vi "write to descriptions.vi"(6 "comment":string, 7 "index":i32, 8 "error in":errorcluster, 9 "Y coords (in moter coordinate)":dbl, 10 "X coords (in moter coordinate)":dbl, 11 "Path of description file":path) -> (0 "error out":errorcluster, 3 "path out":path)   [LabVIEW 2017]
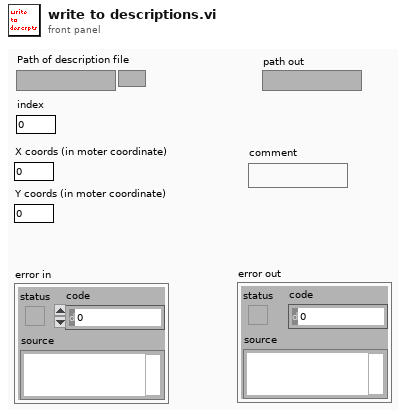
[diagram p1: front panel]
types:
  T1 = enum16{"open", "replace", "create", "open or create", "replace or create", "replace or create with confirmation"}
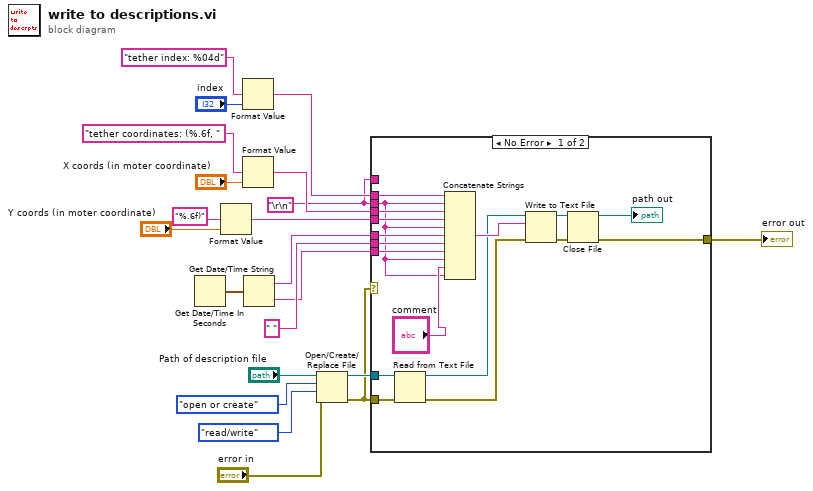
[diagram p0: block diagram]
diagram:
  w1 = "\r\n"
  n1 = Get Date/Time In Seconds() -> (seconds since 1Jan1904=w21:timestamp)
  n2 = Format Value(format string="%.6f)", value (0)="Y coords (in moter coordinate)") -> (output string=w12:string)  [unwired: 1 in]
  n3 = Format Value(format string="tether index: %04d", value (0)="index") -> (output string=w14:string)  [unwired: 1 in]
  n4 = Format Value(format string="tether coordinates: (%.6f, ", value (0)="X coords (in moter coordinate)") -> (output string=w13:string)  [unwired: 1 in]
  n5 = Get Date/Time String(seconds (now)=w21) -> (date string=w11:string, time string=w9:string)  [unwired: 2 in]
  n6 = Open/Create/Replace File(file path (use dialog)="Path of description file", error in="error in", operation (0:open)=T1."open or create", access (0:read/write)=enum16{"read/write", "read-only", "write-only"}."read/write") -> (refnum out=w4:refnum<file>, error out=w3:errorcluster)  [unwired: 2 in, 1 out]
  n7 = case shown="No Error" w3 {
    tunnel: w14 -> [w38 _]
    tunnel: w13 -> [w37 _]
    tunnel: w12 -> [w36 _]
    tunnel: w11 -> [w35 _]
    tunnel: " " -> [w34 _]
    tunnel: w9 -> [w33 _]
    tunnel: w1 -> [w22 _]
    tunnel: w4 -> [w28 _]
    tunnel: w3 -> [w27 w39]
    tunnel: [w24 w39] -> w2
    tunnel: w1 -> [_ _]
    frame No Error {
      n8 = Read from Text File(file (use dialog)=w28, error in=w27) -> (refnum out=w25:refnum<file>, error out=w26:errorcluster)  [unwired: 2 in, 2 out]
      n9 = Concatenate Strings(w38, w22, w37, w36, w22, w35, w34, w33, w22, "comment", w22) -> (w32:string)
      n10 = Write to Text File(file (use dialog)=w25, text=w32, error in=w26) -> (refnum out=w31:refnum<file>, error out=w30:errorcluster)  [unwired: 1 in, 1 out]
      n11 = Close File(refnum=w31, error in=w30) -> (path=→"path out":path, error out=w24:errorcluster)
    }
    frame Error {
    }
  }
  "error out" <- w2
